vi "TxtLog2.vi"(8 "error in (no error)":errorcluster, 9 "trimmed string":string, 10 "CommandString":string, 11 "Byte Stream File in":refnum<file>) -> (0 "error out":errorcluster, 3 "Byte Stream File out":refnum<file>)   [LabVIEW 2017]
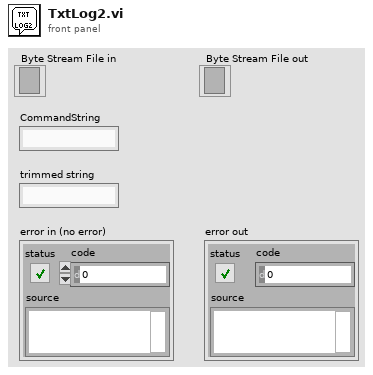
[diagram p1: front panel]
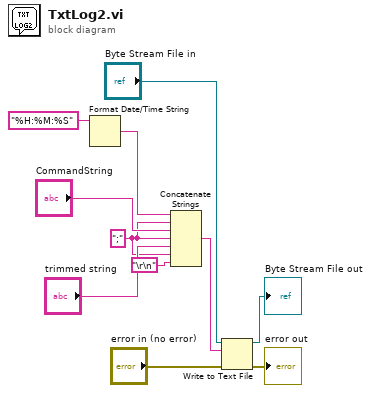
[diagram p0: block diagram]
diagram:
  w1 = ";"
  n1 = Format Date/Time String(time format string (%c)="%H:%M:%S") -> (date/time string=w3:string)  [unwired: 2 in]
  n2 = Concatenate Strings(w3, w1, "CommandString", w1, "trimmed string", w1, "\r\n") -> (w7:string)
  n3 = Write to Text File(file (use dialog)="Byte Stream File in", text=w7, error in="error in (no error)") -> (refnum out=→"Byte Stream File out":refnum<file>, error out=→"error out":errorcluster)  [unwired: 1 in, 1 out]
